vi "Read Program Controls.vi"(8 "error in (no error)":errorcluster, 11 "DROPBEAR_Model_Updating in":refnum<class "DROPBEAR_Model_Updating.lvclass">) -> (0 "error out":errorcluster, 2 "Program Controls":T1={"Frequency KF"=TRUE, "Pinned State KF"=TRUE, "FFT Bounding"=TRUE, "Filter Constants Frequency"={"Measurement Variance"=0.0, "State Variance"=0.0, "Threshold"=0.0}, "Filter Constants Position"={"Measurement Variance"=0.0, "State Variance"=0.0, "Threshold"=0.0}, "Moving Window Size"=0, "Time Series buffer"=0.0, "Record Time Series Data"=FALSE, "Record Moving Window Data"=FALSE, "Record Online Error Metrics "=FALSE, "Record Statistics"=FALSE}, 3 "DROPBEAR_Model_Updating out":refnum<class "DROPBEAR_Model_Updating.lvclass">)   [LabVIEW 2021, in "DROPBEAR_Model_Updating.lvclass"]
uses:
  DROPBEAR_Model_Updating.lvclass
  DROPBEAR_Model_Updating.lvclass/DROPBEAR_Model_Updating.ctl
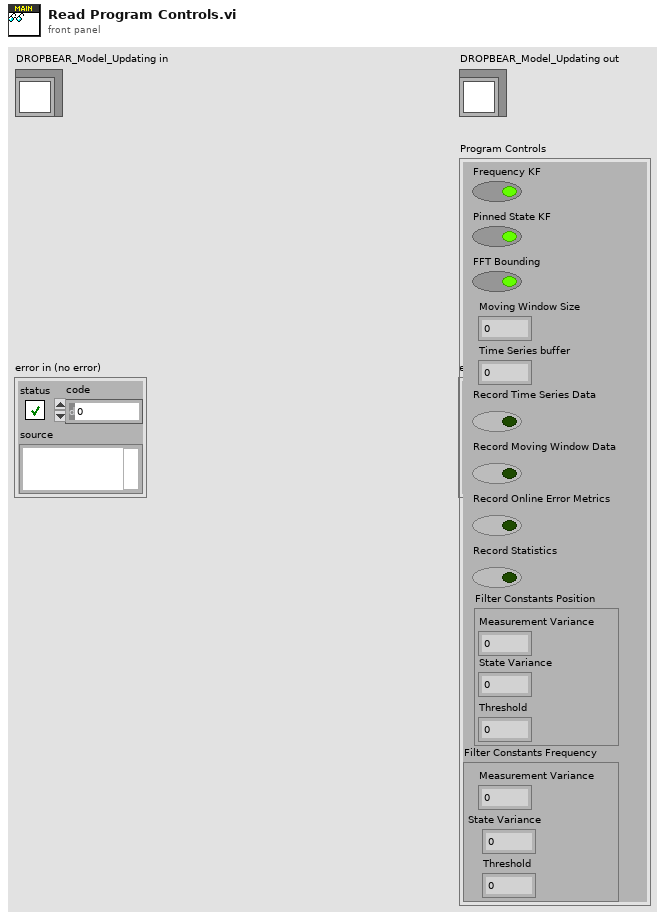
[diagram p1: front panel]
types:
  T1 = cluster{"Frequency KF":bool, "Pinned State KF":bool, "FFT Bounding":bool, "Filter Constants Frequency":cluster{"Measurement Variance":dbl, "State Variance":dbl, "Threshold":dbl}, "Filter Constants Position":cluster{"Measurement Variance":dbl, "State Variance":dbl, "Threshold":dbl}, "Moving Window Size":i32, "Time Series buffer":dbl, "Record Time Series Data":bool, "Record Moving Window Data":bool, "Record Online Error Metrics ":bool, "Record Statistics":bool}
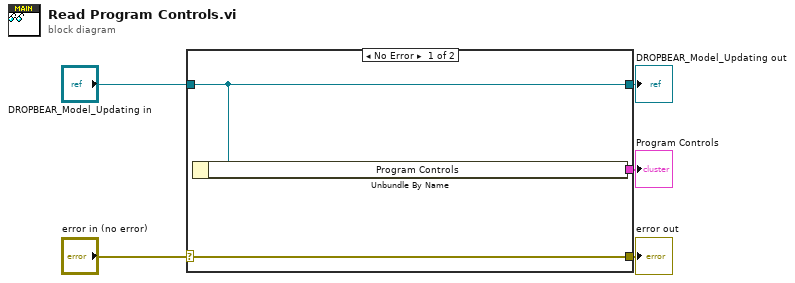
[diagram p0: block diagram]
diagram:
  n1 = case shown="No Error" "error in (no error)" {
    selector: "error in (no error)" -> [w8 w9]
    tunnel: [w8 w9] -> w4
    tunnel: [w7 w10] -> w2
    tunnel: "DROPBEAR_Model_Updating in" -> [w7 w10]
    tunnel: [w6 _] -> w1
    frame No Error {
      n2 = Unbundle By Name(w7) -> ("Program Controls"=w6:T1)
    }
    frame Error {
    }
  }
  "error out" <- w4
  "DROPBEAR_Model_Updating out" <- w2
  "Program Controls" <- w1
